vi "Add Sink.vi"(8 "Log Sink":refnum<class "Log Sink.lvclass">, 9 "Error Queue":refnum<queue>, 10 "Return Queue":refnum<queue>, 11 "Application Logger":refnum<class "Application Logger.lvclass">) -> (0 "error out":errorcluster, 3 "Application Logger out":refnum<class "Application Logger.lvclass">)   [LabVIEW 2019, in "Composed Log.lvlib" / "Application Logger.lvclass"]
uses:
  <vilib>/gpm_packages/@cs/event-logger/Source/Composed Log/Application Logger/Application Logger.lvclass
  <vilib>/gpm_packages/@cs/event-logger/Source/Composed Log/Log Sink/Log Sink.lvclass
  <vilib>/gpm_packages/@cs/event-logger/Source/Composed Log/Application Logger/Application Logger.lvclass/Application Logger.ctl
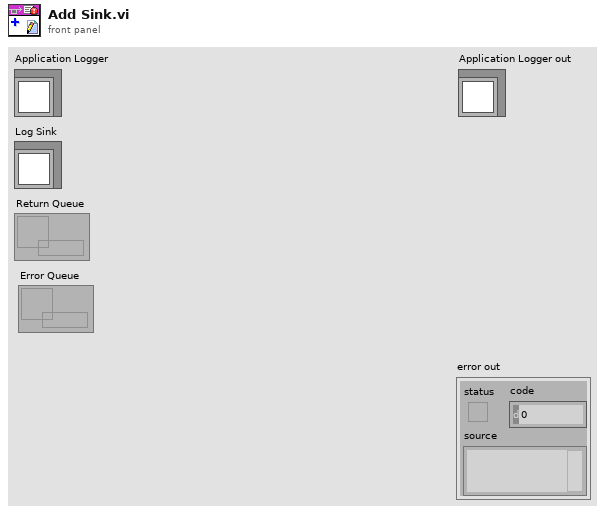
[diagram p1: front panel]
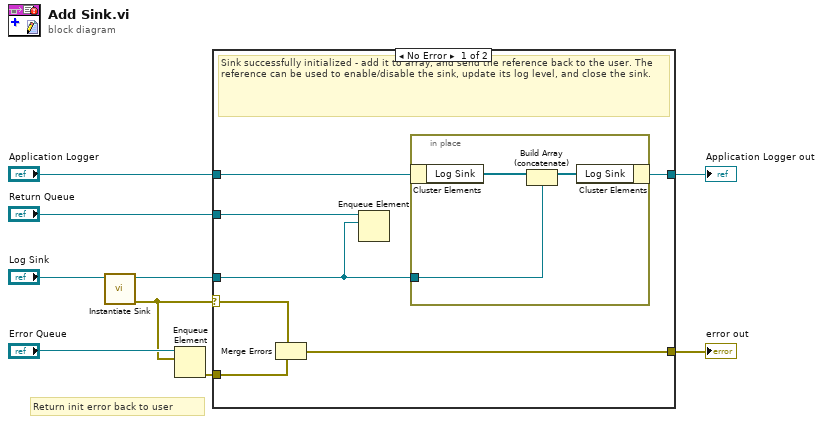
[diagram p0: block diagram]
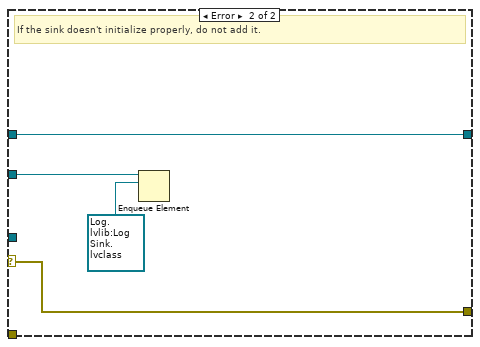
[diagram p2: hidden frame]
diagram:
  # "Return init error back to user"
  n1 = call <vilib>:"Instantiate Sink.vi"("Log Sink in"="Log Sink") -> ("error out"=w2:errorcluster, "Log Sink Reference"=w1:refnum<data-value>)  [unwired: 9 in]
  n2 = Enqueue Element(queue="Error Queue", element=w2) -> (error out=w4:errorcluster)  [unwired: 2 in, 2 out]
  n3 = case shown="No Error" w2 {
    selector: w2 -> [w13 w20]
    tunnel: w1 -> [w12 _]
    tunnel: "Return Queue" -> [w16 w23]
    tunnel: "Application Logger" -> [w11 w21]
    tunnel: [w10 w21] -> w6
    tunnel: [w15 w20] -> w5
    tunnel: w4 -> [w14 _]
    frame No Error {
      # "Sink successfully initialized - add it to array, and send the reference back to the user. The reference can be used to enable/disable the sink, update its log level, and close the sink."
      n4 = Merge Errors(w13, w14) -> (w15:errorcluster)
      n5 = Enqueue Element(queue=w16, element=w12) -> ()  [unwired: 2 in, 3 out]
      n6 = in-place {
        in-place-border: w12 -> [w19]
        n7 = in-place-cluster #1(w11) -> ("Log Sink"=w18:refnum<data-value>[])
        n8 = Build Array (concatenate)(w18, w19) -> (w17:refnum<data-value>[])
        n9 = in-place-cluster #1("Log Sink"=w17) -> (w10:refnum<class "Application Logger.lvclass">)
      }
    }
    frame Error {
      # "If the sink doesn't initialize properly, do not add it."
      n10 = Enqueue Element(queue=w23, element=refnum<data-value> refnum) -> ()  [unwired: 2 in, 3 out]
    }
  }
  "error out" <- w5
  "Application Logger out" <- w6
